vi "Read Pointer.vi"(8 "error in (no error)":errorcluster, 11 "Pointer Base in":refnum<class "Pointer Base.lvclass">) -> (0 "error out":errorcluster, 2 "Pointer":i64, 3 "Pointer Base out":refnum<class "Pointer Base.lvclass">)   [LabVIEW 2020, in "PV Access.lvlib" / "Pointer Base.lvclass"]
uses:
  Pointer Base.lvclass
  Pointer Base.lvclass/Pointer Base.ctl
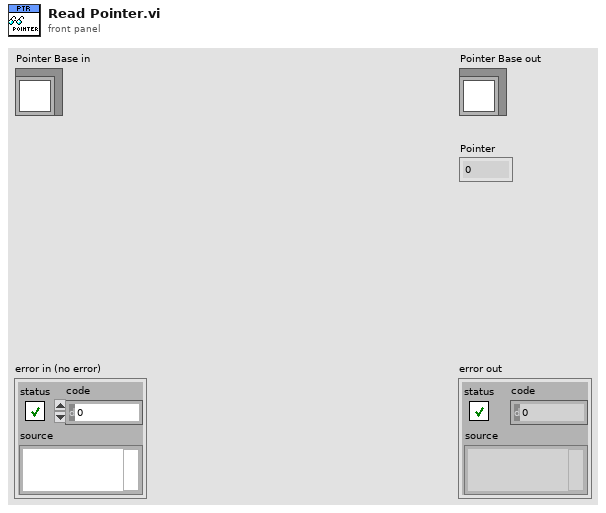
[diagram p1: front panel]
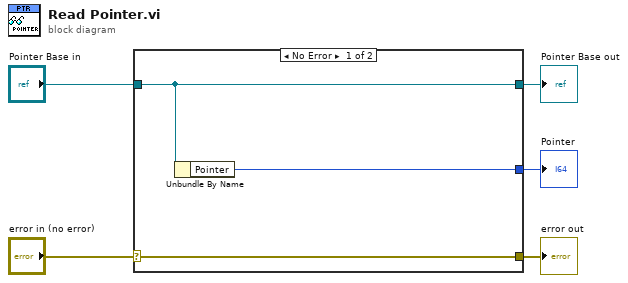
[diagram p0: block diagram]
diagram:
  n1 = case shown="No Error" "error in (no error)" {
    selector: "error in (no error)" -> [w8 w9]
    tunnel: [w8 w9] -> w4
    tunnel: [w7 w10] -> w2
    tunnel: "Pointer Base in" -> [w7 w10]
    tunnel: [w6 _] -> w1
    frame No Error {
      n2 = Unbundle By Name(w7) -> ("Pointer"=w6:i64)
    }
    frame Error {
    }
  }
  "error out" <- w4
  "Pointer Base out" <- w2
  "Pointer" <- w1
